vi "Write Dictionary Element.vi"(8 "error in (no error)":errorcluster, 9 "value":variant, 10 "key":string, 11 "Control Experiment in":refnum<class "Control Experiment.lvclass">) -> (0 "error out":errorcluster, 3 "Control Experiment out":refnum<class "Control Experiment.lvclass">)   [LabVIEW 2020, in "Control Experiment.lvclass"]
uses:
  Control Experiment.lvclass
  Control Experiment.lvclass/Control Experiment.ctl
  <userlib>/_OpenG.lib/dictionary/dictionary.llb/Dictionary Update (by scalar value)__ogtk.vi
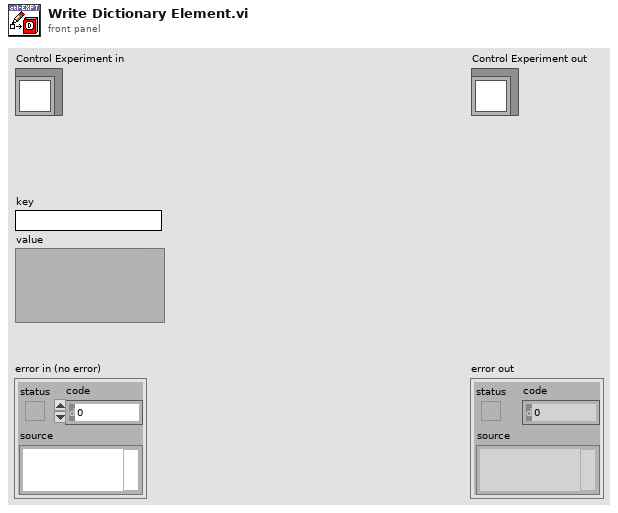
[diagram p1: front panel]
types:
  T1 = typedef "Dictionary Object RefNum__ogtk.ctl" = refnum<k1>
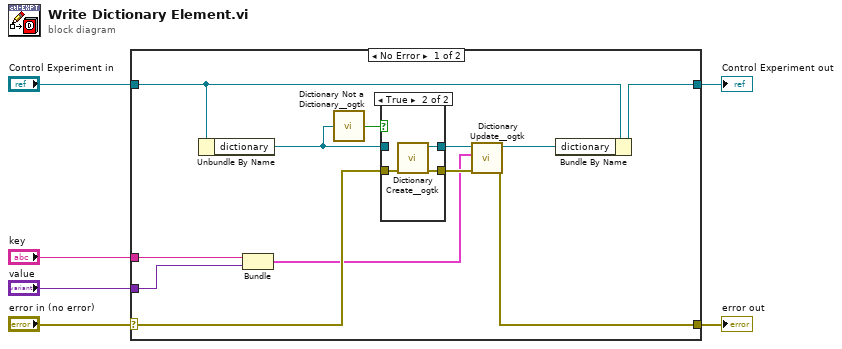
[diagram p0: block diagram]
diagram:
  n1 = case shown="No Error" "error in (no error)" {
    selector: "error in (no error)" -> [w9 w24]
    tunnel: [w13 w24] -> w5
    tunnel: [w18 w25] -> w3
    tunnel: "Control Experiment in" -> [w15 w25]
    tunnel: "key" -> [w17 _]
    tunnel: "value" -> [w16 _]
    frame No Error {
      n2 = Unbundle By Name(w15) -> ("dictionary"=w7:T1)
      n3 = Bundle("key"=w17, "value"=w16) -> (w8:cluster{"key":string, "value":variant})  [unwired: 1 in]
      n4 = call <userlib>:"Dictionary Not a Dictionary__ogtk.vi"("dictionary"=w7) -> ("not a dictionary?"=w11:bool)
      n5 = case shown="True" w11 {
        tunnel: [w20 w23] -> w12
        tunnel: w7 -> [w20 _]
        tunnel: [w19 w22] -> w10
        tunnel: w9 -> [w19 w21]
        frame False {
        }
        frame True {
          n6 = call <userlib>:"Dictionary Create__ogtk.vi"("error in (no error)"=w21) -> ("error out"=w22:errorcluster, "dictionary out"=w23:T1)  [unwired: 9 in]
        }
      }
      n7 = call-poly <userlib>:"Dictionary Update__ogtk.vi"("error in (no error)"=w10, "key-value"=w8, "dictionary"=w12) -> ("error out"=w13:errorcluster, "dictionary out"=w14:T1)  [unwired: 6 in, 1 out]
      n8 = Bundle By Name(cluster=w15, "dictionary"=w14) -> (w18:refnum<class "Control Experiment.lvclass">)
    }
    frame Error {
    }
  }
  "error out" <- w5
  "Control Experiment out" <- w3
